vi "Charger_Get MICS record.vi"(5 "Status Refnum":T2, 6 "error in":errorcluster) -> (0 "error out":errorcluster, 1 "ID":u32 format="%04x", 2 "address":refnum<visa-resource-name>, 3 "MICS Inputs":T1 {"ID" format="%06x"; "chan" min=1 max=10 step=1}, 4 "chan":u16 min=1 max=10 step=1)   [LabVIEW 2020]
doc: "This function gets the MICS Input values from an IPG Status reference."
uses:
  Charger_Status Refnum.ctl
  Drivers/Charger Test Set/Charger_Input Control.ctl
  MICS_Input Control.ctl
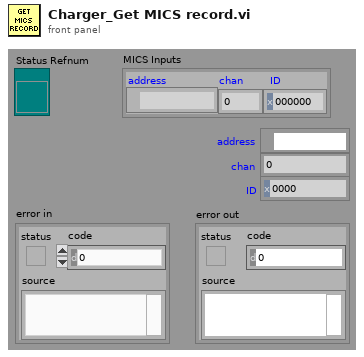
[diagram p1: front panel]
types:
  T1 = typedef "MICS_Input Control.ctl" = cluster{"address":refnum<visa-resource-name>, "chan":u16, "ID":u32}
  T2 = typedef "Charger_Status Refnum.ctl" = refnum<vi>
  T3 = typedef "Charger_Input Control.ctl" = cluster{"address":refnum<visa-resource-name>, "position":i32, "setpoint":dbl}
  T4 = cluster{"MICS ID":u32, "VBAT":dbl, "ChargingState":string, "VBAT Slide":dbl, "Status":string, "TemperatureLevel":dbl, "IPG_ReceivedLevel":dbl, "VBAT Target":dbl, "Charger Setpoint":dbl, "Index":i32, "Ready":bool, "Charger Inputs":T3, "MICS Inputs":cluster{"address":refnum<visa-resource-name>, "chan":u16, "ID":u32}}
  T5 = cluster{"address":refnum<visa-resource-name>, "chan":u16, "ID":u32}
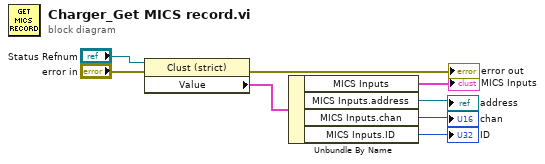
[diagram p0: block diagram]
diagram:
  n1 = property class="Clust (strict)"(reference="Status Refnum", error in="error in") -> (error out=→"error out":errorcluster, "Value"=w8:T4)  [unwired: 1 out]
  n2 = Unbundle By Name(w8) -> ("MICS Inputs"=→"MICS Inputs":T5, "MICS Inputs.address"=→"address":refnum<visa-resource-name>, "MICS Inputs.chan"=→"chan":u16, "MICS Inputs.ID"=→"ID":u32)
